vi "ConvertTextBasedCodeToLabVIEW_CreateMissingTypeList.vi"(11 "Classes":T1[](array[typedef])) -> (3 "MissingItems":T13[](array[typedef]))   [LabVIEW 2012]
uses:
  <resource>/Framework/Providers/Open_GDS/ClassProviders/Common/ConvertTextToLv_SubVIs/ConvertTextBasedCodeToLabVIEW_MissingType.ctl
  <resource>/Framework/Providers/Open_GDS/ClassProviders/Common/ConvertTextToLv_SubVIs/ConvertTextBasedCodeToLabVIEW_MissingTypeIconType.ctl
  <resource>/Framework/Providers/Open_GDS/ClassProviders/Common/String/GDSString_ClassDescriptionType.ctl
  <resource>/Framework/Providers/Open_GDS/ClassProviders/Common/String/GDSString_AccessScopeModifierType.ctl
  <resource>/Framework/Providers/Open_GDS/ClassProviders/Common/String/GDSString_ModifierType.ctl
  <resource>/Framework/Providers/Open_GDS/ClassProviders/Common/String/GDSString_MethodDescriptionType.ctl
  <resource>/Framework/Providers/Open_GDS/ClassProviders/Common/CommonVIs/CommonVIs_AttributeType.ctl
  <resource>/Framework/Providers/Open_GDS/ClassProviders/Common/CommonVIs/CommonVIs_AttributeDataType.ctl
  <resource>/Framework/Providers/Open_GDS/ClassProviders/Common/CommonVIs/CommonVIs_PropertyType.ctl
  <resource>/Framework/Providers/Open_GDS/ClassProviders/Common/String/GDSString_ClassParentType.ctl
  <resource>/Framework/Providers/Open_GDS/ClassProviders/Common/String/GDSString_ClassType.ctl
  <resource>/Framework/Providers/Open_GDS/ClassProviders/Common/String/GDSString_ClassOwnerType.ctl
  <resource>/Framework/Providers/Open_GDS/ClassProviders/Common/CommonVIs/CommonVIs_EnumType.ctl
  <resource>/Framework/Providers/Open_GDS/ClassProviders/Common/CommonVIs/CommonVIs_StructType.ctl
  <resource>/Framework/Providers/Open_GDS/ClassProviders/Common/ConvertTextToLv_SubVIs/ConvertTextBasedCodeToLabVIEW_MissingTypeOptions.ctl
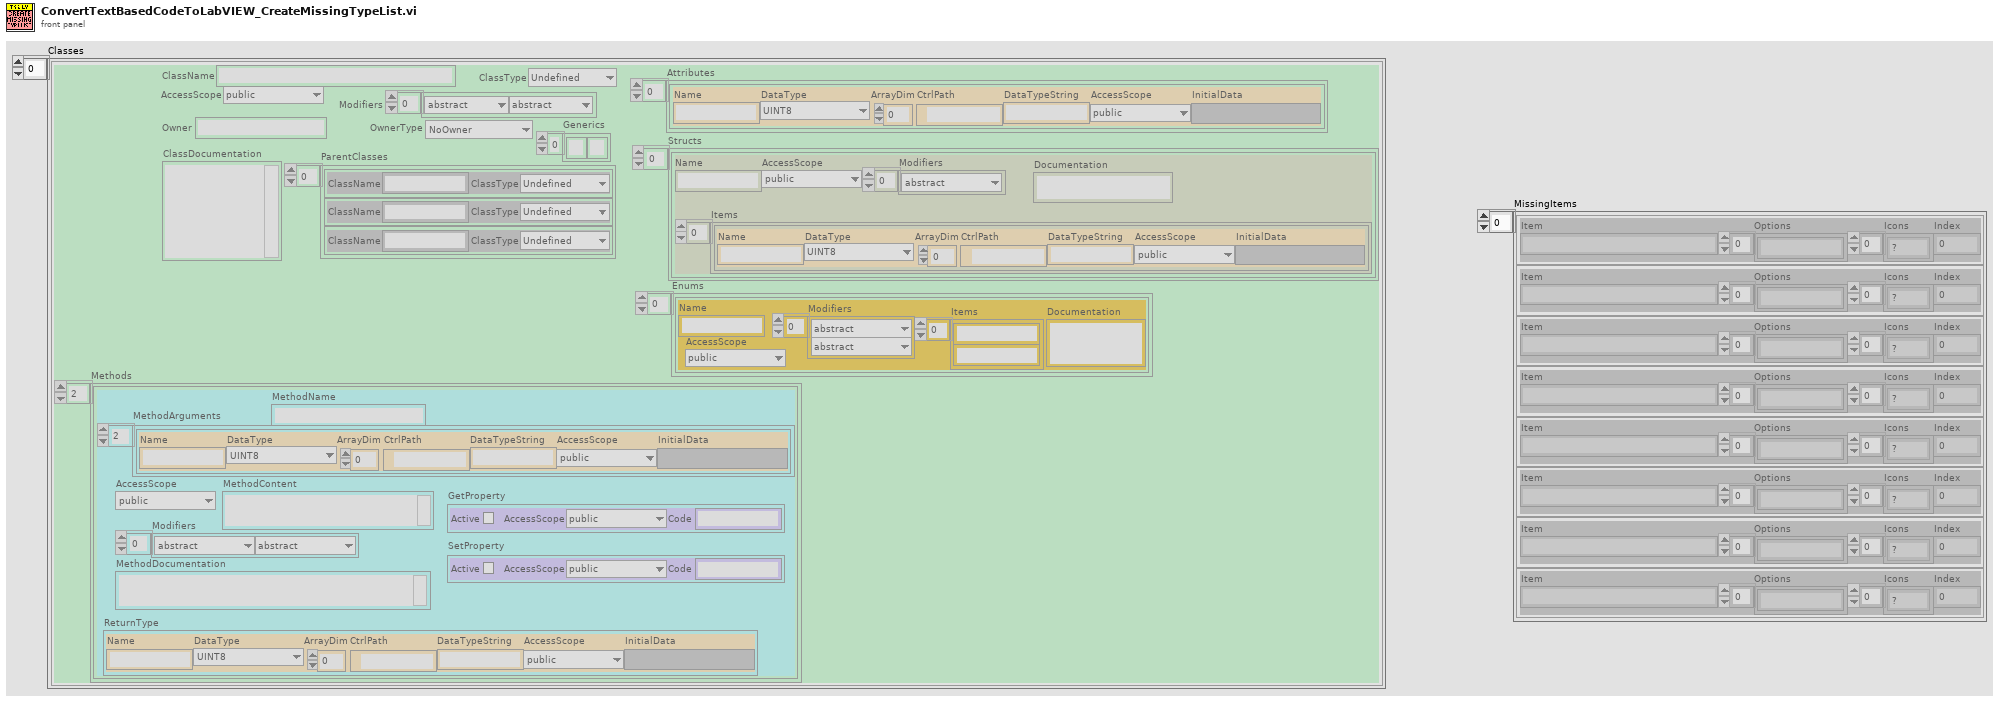
[diagram p1: front panel]
types:
  T1 = typedef "GDSString_ClassDescriptionType.ctl" = cluster{"ClassName":string, "AccessScope":T2, "Modifiers":T3[], "ClassDocumentation":string, "Methods":T4[], "ParentClasses":T8[], "ClassType":T9, "Owner":string, "OwnerType":T10, "Generics":string[], "Attributes":T5[], "Enums":T11[], "Structs":T12[]}
  T2 = typedef "GDSString_AccessScopeModifierType.ctl" = enum16{"public", "private", "protected", "internal"}
  T3 = typedef "GDSString_ModifierType.ctl" = enum16{"abstract", "static", "final", "synchronized", "strictfp", "async", "const", "event", "extern", "new", "native ", "override", "partial", "readonly", "sealed", "unsafe", "virtual", "volatile"}
  T4 = typedef "GDSString_MethodDescriptionType.ctl" = cluster{"ReturnType":T5, "MethodName":string, "AccessScope":T2, "Modifiers":T3[], "MethodDocumentation":string, "MethodContent":string, "MethodArguments":T5[], "GetProperty":T7, "SetProperty":T7}
  T5 = typedef "CommonVIs_AttributeType.ctl" = cluster{"Name":string, "DataType":T6, "ArrayDim":i32, "CtrlPath":path, "DataTypeString":string, "AccessScope":T2, "InitialData":variant}
  T6 = typedef "CommonVIs_AttributeDataType.ctl" = enum16{"UINT8", "INT8", "UINT16", "INT16", "UINT32", "INT32", "UINT64", "INT64", "SGL", "DBL", "EXT", "CSG", "CDB", "CXT", "TimeStamp", "STRING", "PATH", "BOOL", "ENUM", "RefNum", "VIRefNum", "LabVIEW Class", "Cluster", "Variant", "TypeDef", "Waveform", "LabVIEW Object", "Other", "void"}
  T7 = typedef "CommonVIs_PropertyType.ctl" = cluster{"Active":bool, "AccessScope":T2, "Code":string}
  T8 = typedef "GDSString_ClassParentType.ctl" = cluster{"ClassName":string, "ClassType":T9}
  T9 = typedef "GDSString_ClassType.ctl" = enum16{"Undefined", "Class", "Interface"}
  T10 = typedef "GDSString_ClassOwnerType.ctl" = enum16{"NoOwner", "Class", "Package/NameSpace"}
  T11 = typedef "CommonVIs_EnumType.ctl" = cluster{"Name":string, "AccessScope":T2, "Modifiers":T3[], "Items":string[], "Documentation":string}
  T12 = typedef "CommonVIs_StructType.ctl" = cluster{"Name":string, "AccessScope":T2, "Modifiers":T3[], "Items":T5[], "Documentation":string}
  T13 = typedef "ConvertTextBasedCodeToLabVIEW_MissingType.ctl" = cluster{"Item":string, "Options":string[], "Icons":T14[], "Index":i32}
  T14 = typedef "ConvertTextBasedCodeToLabVIEW_MissingTypeIconType.ctl" = enum16{"?", "Add", "Delete"}
  T15 = typedef "ConvertTextBasedCodeToLabVIEW_MissingTypeOptions.ctl" = enum16{"Select action to handle missing type", "Create stub code as class", "Create stub code as interface by VI Server", "Remove dependency to this type"}
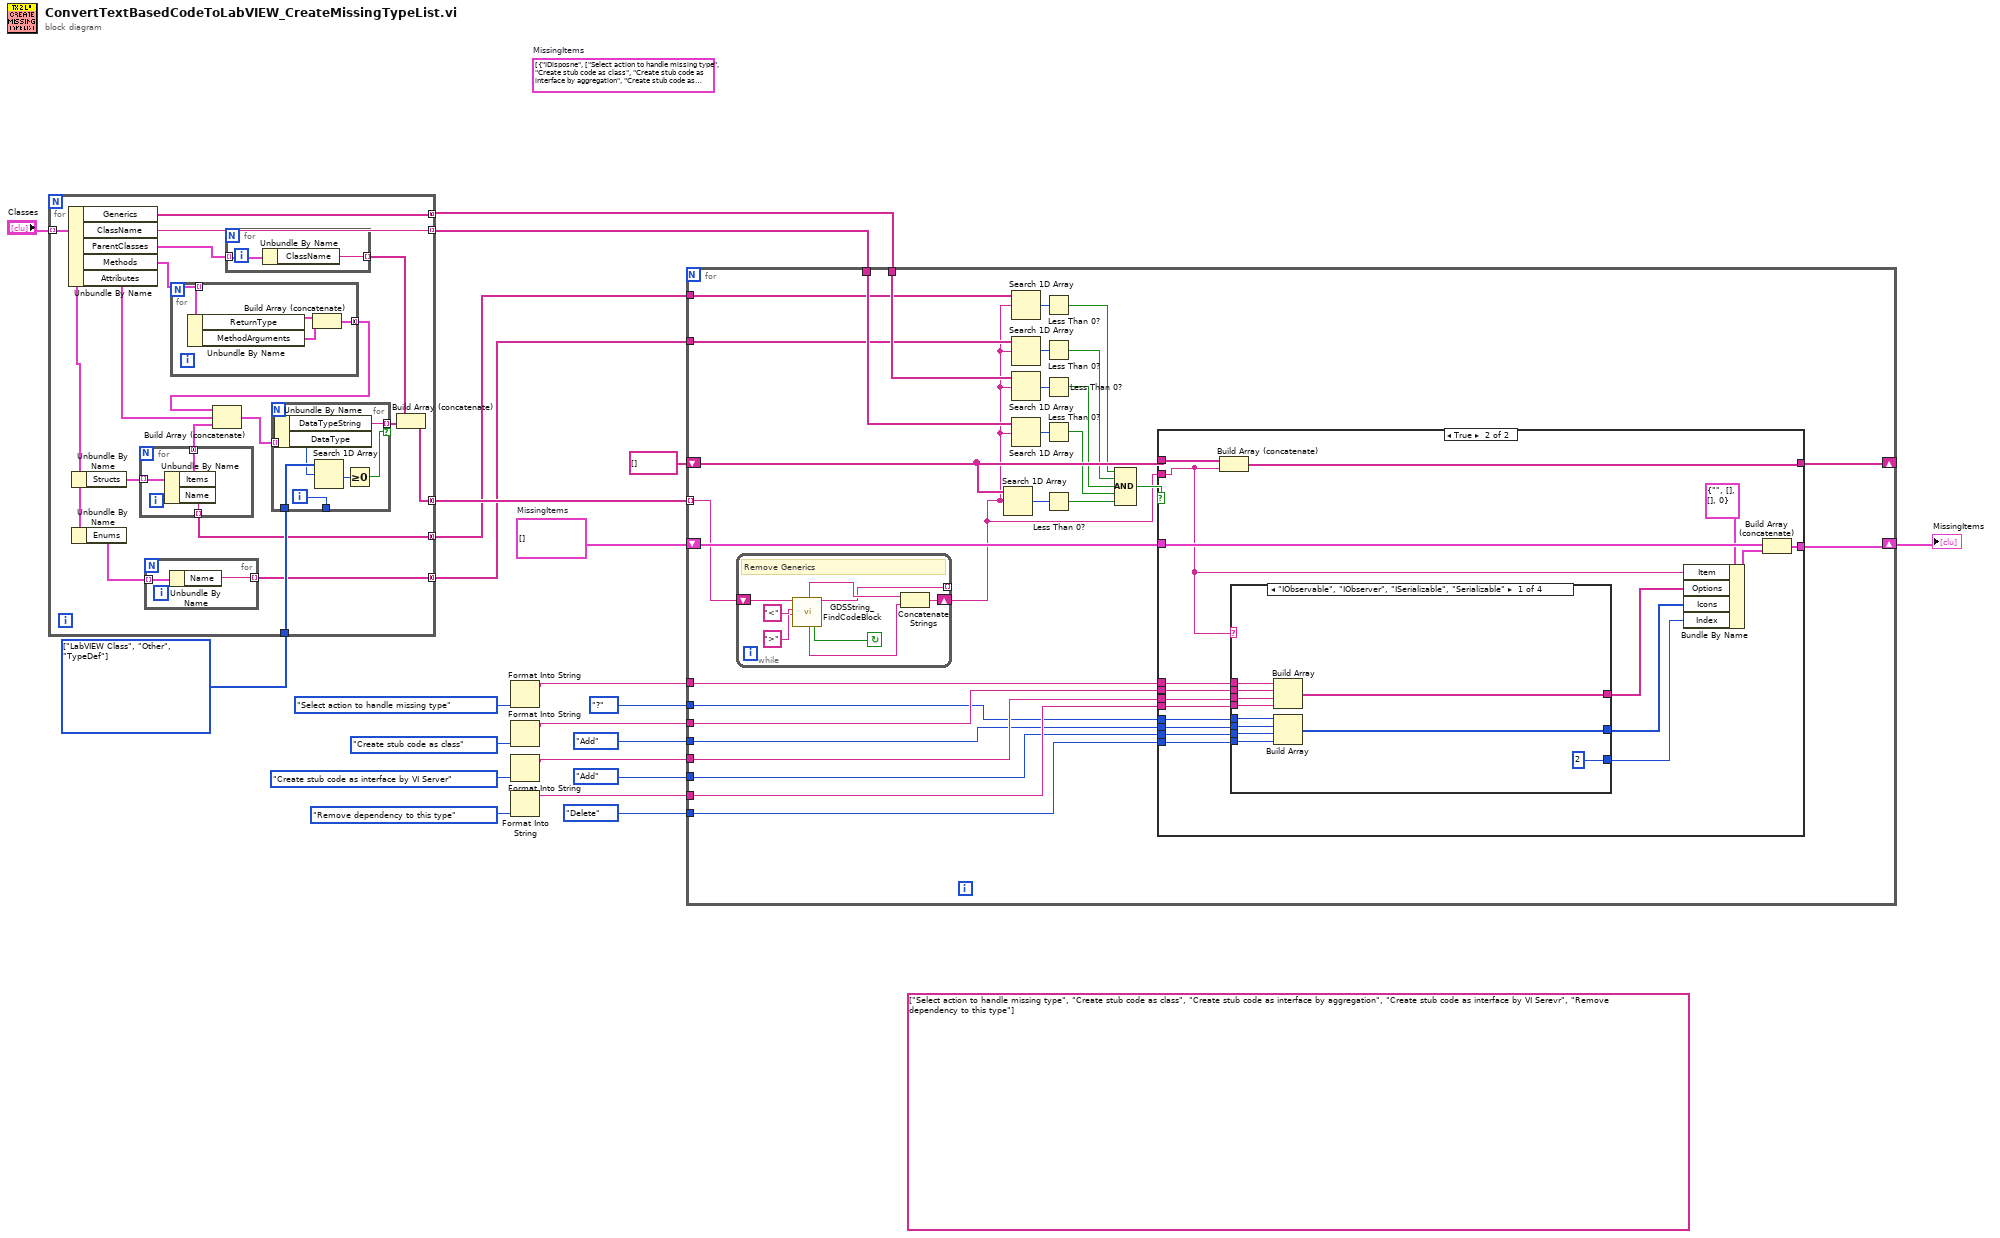
[diagram p0: block diagram]
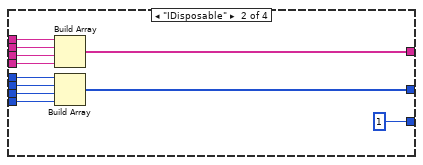
[diagram p3: hidden frame]
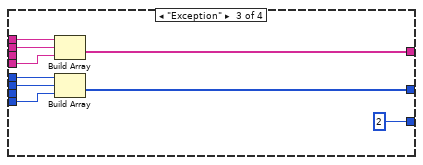
[diagram p4: hidden frame]
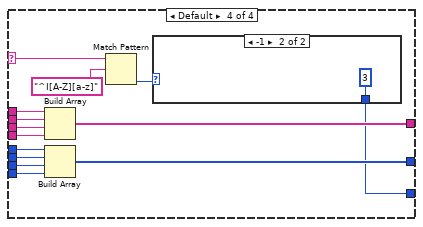
[diagram p5: hidden frame]
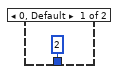
[diagram p6: hidden frame]
diagram:
  (unwired) string[] ["Select action to handle missing type", "Create stub code as class", "Create stub code as interface by aggregation", "Create stub code as interface by VI Serevr", "Remove dependency to this type"] ("Options")
  w16 = T13[] []  # MissingItems
  (unwired) T13[] [{"Item"="IDisposne", "Options"=["Select action to handle missing type", "Create stub code as class", "Create stub code as interface by aggregation", "Create stub code as interface by VI Serevr", "Remove dependency to this type"], "Icons"=[enum."?", enum."Add", enum."Add", enum."Add", enum."Delete"], "Index"=0}, {"Item"="IInterafceXXX", "Options"=["Select action to handle missing type", "Create stub code as class", "Create stub code as interface by VI Serevr", "Remove dependency to this type"], "Icons"=[enum."?", enum."Add", enum."Add", enum."Delete"], "Index"=1}, {"Item"="Something Something", "Options"=["Select action to handle missing type", "Create stub code as class", "Remove dependency to this type"], "Icons"=[enum."?", enum."Add", enum."Delete"], "Index"=2}, {"Item"="Something Something", "Options"=["Select action to handle missing type", "Create stub code as class", "Remove dependency to this type"], "Icons"=[enum."?", enum."Add", enum."Delete"], "Index"=2}, {"Item"="Something Something", "Options"=["Select action to handle missing type", "Create stub code as class", "Remove dependency to this type"], "Icons"=[enum."?", enum."Add", enum."Delete"], "Index"=2}, {"Item"="Something Something", "Options"=["Select action to handle missing type", "Create stub code as class", "Remove dependency to this type"], "Icons"=[enum."?", enum."Add", enum."Delete"], "Index"=2}, {"Item"="Something Something", "Options"=["Select action to handle missing type", "Create stub code as class", "Remove dependency to this type"], "Icons"=[enum."?", enum."Add", enum."Delete"], "Index"=2}, {"Item"="Something Something", "Options"=["Select action to handle missing type", "Create stub code as class", "Remove dependency to this type"], "Icons"=[enum."?", enum."Add", enum."Delete"], "Index"=2}]  # MissingItems
  w19 = T6[] [enum."LabVIEW Class", enum."Other", enum."TypeDef"] items=["UINT8", "INT8", "UINT16", "INT16", "UINT32", "INT32", "UINT64", "INT64", "SGL", "DBL", "EXT", "CSG", "CDB", "CXT", "TimeStamp", "STRING", "PATH", "BOOL", "ENUM", "RefNum", "VIRefNum", "LabVIEW Class", "Cluster", "Variant", "TypeDef", "Waveform", "LabVIEW Object", "Other", "void"] ("1D array")
  n1 = for {
    tunnel: "Classes" -> [w25] mode=indexing
    tunnel: [w39] -> w21 mode=indexing
    tunnel: [w27] -> w20 mode=concatenating
    tunnel: w19 -> [w29]
    tunnel: [w35] -> w22 mode=concatenating
    tunnel: [w26] -> w10 mode=concatenating
    tunnel: [w23] -> w9 mode=concatenating
    n2 = Unbundle By Name(w25) -> ("Generics"=w35:string[], "ClassName"=w39:string, "ParentClasses"=w38:T8[], "Methods"=w37:T4[], "Attributes"=w34:T5[])
    n3 = Unbundle By Name(w25) -> ("Structs"=w32:T12[])
    n4 = Unbundle By Name(w25) -> ("Enums"=w24:T11[])
    n5 = for {
      tunnel: w32 -> [w51] mode=indexing
      tunnel: [w50] -> w31 mode=concatenating
      tunnel: [w49] -> w26 mode=indexing
      n6 = Unbundle By Name(w51) -> ("Items"=w50:T5[], "Name"=w49:string)
    }
    n7 = for {
      tunnel: w24 -> [w41] mode=indexing
      tunnel: [w40] -> w23 mode=indexing
      n8 = Unbundle By Name(w41) -> ("Name"=w40:string)
    }
    n9 = for {
      tunnel: w37 -> [w55] mode=indexing
      tunnel: [w52] -> w33 mode=concatenating
      n10 = Unbundle By Name(w55) -> ("ReturnType"=w54:T5, "MethodArguments"=w53:T5[])
      n11 = Build Array (concatenate)(w54, w53) -> (w52:T5[])
    }
    n12 = Build Array (concatenate)(w33, w34, w31) -> (w30:T5[])
    n13 = for {
      tunnel: w38 -> [w57] mode=indexing
      tunnel: [w56] -> w36 mode=indexing
      n14 = Unbundle By Name(w57) -> ("ClassName"=w56:string)
    }
    n15 = for {
      tunnel: w30 -> [w48] mode=indexing
      tunnel: w29 -> [w47]
      tunnel: [w44] -> w28 mode=indexing if=w43
      tunnel: [w42] -> _
      i -> [w42]
      n16 = Unbundle By Name(w48) -> ("DataTypeString"=w44:string, "DataType"=w46:T6)
      n17 = Search 1D Array(1D array=w47, element=w46) -> (index of element=w45:i32)  [unwired: 1 in]
      n18 = Greater Or Equal To 0?(x=w45) -> (x >= 0?=w43:bool)
    }
    n19 = Build Array (concatenate)(w36, w28) -> (w27:string[])
  }
  n20 = Format Into String(ConvertTextBasedCodeToLabVIEW_MissingTypeOptions."Select action to handle missing type") -> (resulting string=w4:string)  [unwired: 3 in, 1 out]
  n21 = Format Into String(ConvertTextBasedCodeToLabVIEW_MissingTypeOptions."Create stub code as class") -> (resulting string=w1:string)  [unwired: 3 in, 1 out]
  n22 = Format Into String(ConvertTextBasedCodeToLabVIEW_MissingTypeOptions."Create stub code as interface by VI Server") -> (resulting string=w5:string)  [unwired: 3 in, 1 out]
  n23 = Format Into String(ConvertTextBasedCodeToLabVIEW_MissingTypeOptions."Remove dependency to this type") -> (resulting string=w7:string)  [unwired: 3 in, 1 out]
  n24 = for {
    tunnel: w20 -> [w65] mode=indexing
    shift-right: [w82] -> _
    shift-left: string[] [] -> [w83]
    tunnel: w21 -> [w81]
    tunnel: w22 -> [w78]
    shift-right: [w74] -> w15
    shift-left: w16 -> [w75]
    tunnel: w4 -> [w73]
    tunnel: w1 -> [w72]
    tunnel: w5 -> [w71]
    tunnel: w7 -> [w70]
    tunnel: ConvertTextBasedCodeToLabVIEW_MissingTypeIconType."?" ("Icon") -> [w69]
    tunnel: ConvertTextBasedCodeToLabVIEW_MissingTypeIconType."Add" ("Icon") -> [w68]
    tunnel: ConvertTextBasedCodeToLabVIEW_MissingTypeIconType."Add" ("Icon") -> [w67]
    tunnel: ConvertTextBasedCodeToLabVIEW_MissingTypeIconType."Delete" ("Icon") -> [w66]
    tunnel: w10 -> [w62]
    tunnel: w9 -> [w61]
    n25 = while {
      shift-right: [w88] -> w60
      shift-left: w65 -> [w94]
      tunnel: [w87] -> _ mode=indexing
      stop <- w91 continue-if-true
      # "Remove Generics"
      n26 = call <resource>:"GDSString_FindCodeBlock.vi"("Text"=w94, "CodeBlockStartCharacter( { )"="<", "CodeBlockEndCharacter( } )"=">") -> ("TextBeforeBlock"=w90:string, "TextAfterBlock"=w89:string, "found"=w91:bool, "BlockText"=w87:string)  [unwired: 8 in, 5 out]
      n27 = Concatenate Strings(w90, w89) -> (w88:string)
    }
    n28 = Search 1D Array(1D array=w83, element=w60) -> (index of element=w86:i32)  [unwired: 1 in]
    n29 = Search 1D Array(1D array=w62, element=w60) -> (index of element=w64:i32)  [unwired: 1 in]
    n30 = Search 1D Array(1D array=w61, element=w60) -> (index of element=w63:i32)  [unwired: 1 in]
    n31 = Search 1D Array(1D array=w78, element=w60) -> (index of element=w77:i32)  [unwired: 1 in]
    n32 = Search 1D Array(1D array=w81, element=w60) -> (index of element=w80:i32)  [unwired: 1 in]
    n33 = Less Than 0?(x=w64) -> (x < 0?=w58:bool)
    n34 = Less Than 0?(x=w63) -> (x < 0?=w59:bool)
    n35 = Less Than 0?(x=w77) -> (x < 0?=w76:bool)
    n36 = Less Than 0?(x=w80) -> (x < 0?=w79:bool)
    n37 = Less Than 0?(x=w86) -> (x < 0?=w84:bool)
    n38 = Compound Arithmetic op=AND(w58, w59, w76, w79, w84) -> (w85:bool)
    n39 = case shown="True" w85 {
      tunnel: w83 -> [w96 w114]
      tunnel: w60 -> [_ w108]
      tunnel: [w96 w113] -> w82
      tunnel: w75 -> [w95 w112]
      tunnel: [w95 w111] -> w74
      tunnel: w73 -> [_ w107]
      tunnel: w72 -> [_ w106]
      tunnel: w71 -> [_ w105]
      tunnel: w70 -> [_ w104]
      tunnel: w69 -> [_ w103]
      tunnel: w68 -> [_ w102]
      tunnel: w67 -> [_ w101]
      tunnel: w66 -> [_ w100]
      frame False {
      }
      frame True {
        n40 = Build Array (concatenate)(w114, w108) -> (w113:string[])
        n41 = case shown="\"IObservable\", \"IObserver\", \"ISerializable\", \"Serializable\"" w108 {
          selector: w108 -> [_ _ _ w159]
          tunnel: w107 -> [w125 w136 w145 w156]
          tunnel: w106 -> [w124 w135 w144 w155]
          tunnel: w105 -> [w123 w134 _ w154]
          tunnel: w104 -> [w122 w133 w143 w153]
          tunnel: w103 -> [w121 w132 w142 w149]
          tunnel: w102 -> [w120 w131 w141 w150]
          tunnel: w101 -> [w119 w130 _ w151]
          tunnel: w100 -> [w118 w129 w140 w152]
          tunnel: [w117 w128 w139 w148] -> w99
          tunnel: [w116 w127 w138 w147] -> w98
          tunnel: [2 ("InitialIndex") 1 ("InitialIndex") 2 ("InitialIndex") w146] -> w97
          frame "IObservable", "IObserver", "ISerializable", "Serializable" {
            n42 = Build Array(w125, w124, w123, w122) -> (w117:string[])
            n43 = Build Array(w121, w120, w119, w118) -> (w116:T14[])
          }
          frame "IDisposable" {
            n44 = Build Array(w136, w135, w134, w133) -> (w128:string[])
            n45 = Build Array(w132, w131, w130, w129) -> (w127:T14[])
          }
          frame "Exception" {
            n46 = Build Array(w145, w144, w143) -> (w139:string[])
            n47 = Build Array(w142, w141, w140) -> (w138:T14[])
          }
          frame Default {
            n48 = Build Array(w156, w155, w154, w153) -> (w148:string[])
            n49 = Build Array(w149, w150, w151, w152) -> (w147:T14[])
            n50 = Match Pattern(string=w159, regular expression="^I[A-Z][a-z]") -> (offset past match=w157:i32)  [unwired: 1 in, 3 out]
            n51 = case shown="-1" w157 {
              tunnel: [2 ("InitialIndex") 3 ("InitialIndex")] -> w146
              frame 0, Default {
              }
              frame -1 {
              }
            }
          }
        }
        n52 = Bundle By Name(cluster=T13 {"Item"="", "Options"=[], "Icons"=[], "Index"=0} ("Cluster"), "Item"=w108, "Options"=w99, "Icons"=w98, "Index"=w97) -> (w109:T13)
        n53 = Build Array (concatenate)(w112, w109) -> (w111:T13[])
      }
    }
  }
  "MissingItems" <- w15
